vi "ConvertWaterMixValve4Calibration.vi"(8 "Water Mix Valve":u16(ring) items=["A1", "A2", "A3", "A4", "B1", "B2", "B3", "B4", "B5", "B6", "B7", "B8", "A5", "A6", "A7", "A8"], 9 "Ctr Water Valve":u16(ring) items=["A1", "A2", "A3", "A4", "B1", "B2", "B3", "B4", "B5", "B6", "B7", "B8", "A5", "A6", "A7", "A8"], 11 "Calibration Refs":T2) -> (0 "Water Calibration?":bool[](array[boolean]), 1 "PressList":u8[](array[numeric]), 2 "RatioList":dbl[](array[numeric]), 3 "Valve Signal Array":T1(array[cluster]))   [LabVIEW 2016]
uses:
  <vilib>/imath/engines/lvmath/Plug In/_Char/NIMS_CH_character datatype.ctl
  <vilib>/imath/engines/lvmath2/RunTimeEngine/VariableToken/Support/NIMS_Vector Boolean Index to I32 Index.vi
  <vilib>/imath/engines/lvmath2/RunTimeEngine/IndexRead/NIMS V(V).vi
  <instcachedir>/0/NIMS V(V)_298D9CB7BFEB42B8BC8D9C3C28AE8C70.lvgen/NIMS V(V)_298D9CB7BFEB42B8BC8D9C3C28AE8C70_001.vi
  <vilib>/imathl/engines/lvmath/Functions/Error Handling/Create Error.vi
  <instcachedir>/0/NIMS V(V)_298D9CB7BFEB42B8BC8D9C3C28AE8C70.lvgen/NIMS V(V)_298D9CB7BFEB42B8BC8D9C3C28AE8C70_002.vi
  <vilib>/imath/engines/lvmath2/RunTimeEngine/IndexReplace/NIMS V(V)=V.vi
  <instcachedir>/0/NIMS V(V)=V_BE8E060C6E1D4A13ABFD54A163A3AD30.lvgen/NIMS V(V)=V_BE8E060C6E1D4A13ABFD54A163A3AD30_000.vi
  <vilib>/imath/engines/lvmath2/RunTimeEngine/ErrorHandling/NIMS_Create Error From Enums.vi
  <vilib>/imath/engines/lvmath2/RunTimeEngine/BuiltInFunctions/findnz/NIMS_[1o]_findnz(GRowV).vi
  <instcachedir>/0/NIMS_[1o]_findnz(GRowV)_656056C849EF4762B1F0843BDDDEF2FF.lvgen/NIMS_[1o]_findnz(GRowV)_656056C849EF4762B1F0843BDDDEF2FF_000.vi
  <vilib>/imath/engines/lvmath/Plug In/_Char/NIMS_CH_Character RV to String.vi
  <vilib>/imath/engines/lvmath2/RunTimeEngine/BuiltInFunctions/length/NIMS_length(GV).vi
  <instcachedir>/0/NIMS_length(GV)_08A3D13377FD4E4B96F5795FBF3698FA.lvgen/NIMS_length(GV)_08A3D13377FD4E4B96F5795FBF3698FA_002.vi
  <vilib>/imath/engines/lvmath2/RunTimeEngine/BuiltInFunctions/random/NIMS_random.vi
  <vilib>/imath/engines/lvmath2/RunTimeSupport/NIMS_Error if Not Equal.vi
  <instcachedir>/0/NIMS_Error if Not Equal_EBDB539BFBF84063AF66BAE64AA6DE72.lvgen/NIMS_Error if Not Equal_EBDB539BFBF84063AF66BAE64AA6DE72_002.vi
  <vilib>/imath/engines/lvmath2/RunTimeEngine/IndexRead/NIMS V(M).vi
  <instcachedir>/0/NIMS V(M)_9C733378D59448EDB8B370EA0429D12A.lvgen/NIMS V(M)_9C733378D59448EDB8B370EA0429D12A_002.vi
  <instcachedir>/0/NIMS V(M)_9C733378D59448EDB8B370EA0429D12A.lvgen/NIMS V(M)_9C733378D59448EDB8B370EA0429D12A_001.vi
  <vilib>/imath/engines/lvmath2/RunTimeEngine/IndexReplace/NIMS V(V)=M.vi
  <instcachedir>/0/NIMS V(V)=M_4E1E70A83EF34EDC81D1F331EC25431D.lvgen/NIMS V(V)=M_4E1E70A83EF34EDC81D1F331EC25431D_001.vi
  <instcachedir>/0/NIMS V(M)_9C733378D59448EDB8B370EA0429D12A.lvgen/NIMS V(M)_9C733378D59448EDB8B370EA0429D12A_000.vi
  <instcachedir>/0/NIMS V(V)=M_4E1E70A83EF34EDC81D1F331EC25431D.lvgen/NIMS V(V)=M_4E1E70A83EF34EDC81D1F331EC25431D_002.vi
  <vilib>/imath/engines/lvmath2/RunTimeEngine/NodeEndStatement/NIMS_NodeEndStatement_Output.vi
  <instcachedir>/0/NIMS_NodeEndStatement_Output_53EC0D466D134D7ABD903AC30B43404B.lvgen/NIMS_NodeEndStatement_Output_53EC0D466D134D7ABD903AC30B43404B_013.vi
  <instcachedir>/0/NIMS_NodeEndStatement_Output_53EC0D466D134D7ABD903AC30B43404B.lvgen/NIMS_NodeEndStatement_Output_53EC0D466D134D7ABD903AC30B43404B_012.vi
  <instcachedir>/0/NIMS_NodeEndStatement_Output_53EC0D466D134D7ABD903AC30B43404B.lvgen/NIMS_NodeEndStatement_Output_53EC0D466D134D7ABD903AC30B43404B_011.vi
  <instcachedir>/0/NIMS_NodeEndStatement_Output_53EC0D466D134D7ABD903AC30B43404B.lvgen/NIMS_NodeEndStatement_Output_53EC0D466D134D7ABD903AC30B43404B_005.vi
  <vilib>/imath/engines/lvmath2/RunTimeEngine/ErrorHandling/NIMS_Finalize Error.vi
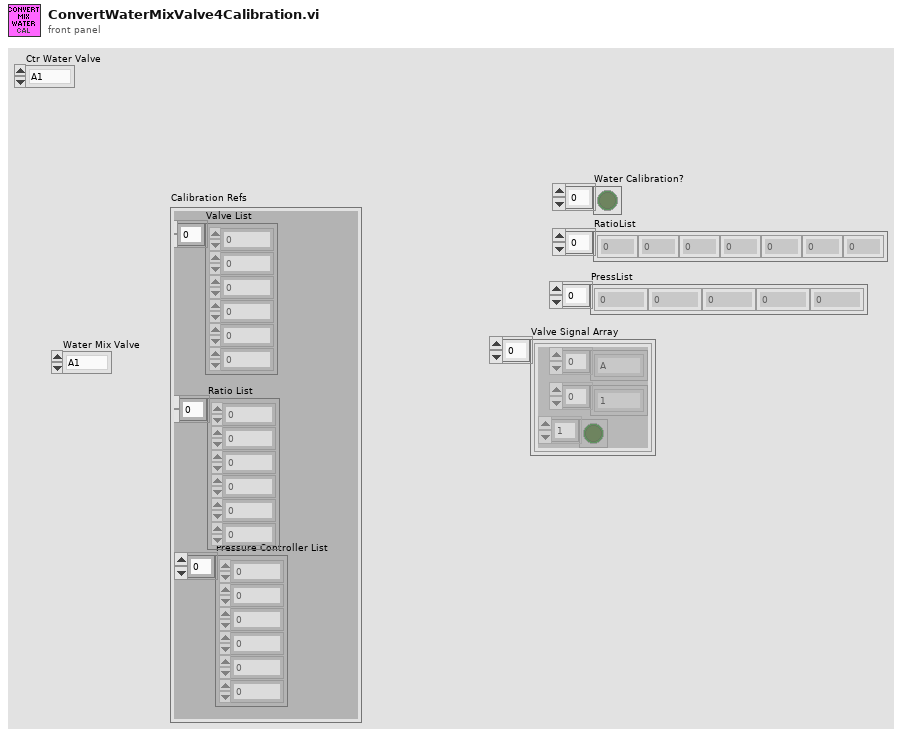
[diagram p1: front panel]
types:
  T1 = cluster{enum16{"A", "B", "C"}[], enum16{"1", "2", "3", "4", "5", "6", "7", "8"}[], bool[]}[]
  T2 = cluster{"Pressure Controller List":u8[], "Ratio List":dbl[], "Valve List":u16[]}
  T3 = cluster{"Flowboards":enum16{"A", "B", "C"}[], "Channels":enum16{"1", "2", "3", "4", "5", "6", "7", "8"}[], "States":bool[]}[]
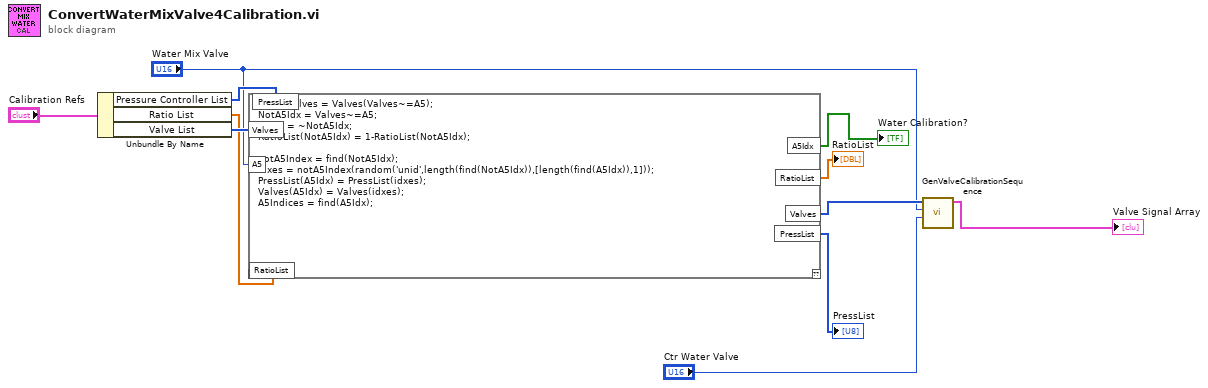
[diagram p0: block diagram]
diagram:
  n1 = Unbundle By Name("Calibration Refs") -> ("Pressure Controller List"=w10:u8[], "Ratio List"=w8:dbl[], "Valve List"=w9:u16[])
  n2 = mathscript code="NotA5Valves = Valves(Valves~=A5);\nNotA5Idx = Valves~=A5;\nA5Idx = ~NotA5Idx;\nRatioList(NotA5Idx) = 1-RatioList(NotA5Idx);\n\nnotA5Index = find(NotA5Idx);\nidxes = notA5Index(random('unid',length(find(NotA5Idx)),[length(find(A5Idx)),1]));\nPressList(A5Idx) = PressList(idxes);\nValves(A5Idx) = Valves(idxes);\nA5Indices = find(A5Idx);"("A5"="Water Mix Valve", "Valves"=w9, "PressList"=w10, "RatioList"=w8) -> ("RatioList"=→"RatioList":dbl[], "Valves"=w4:u16[], "PressList"=→"PressList":u8[], "A5Idx"=→"Water Calibration?":bool[])  [unwired: 1 in, 1 out]
  n3 = call "GenValveCalibrationSequence.vi"("Ctr Odor Valve"="Ctr Water Valve", "Water Mix Valve"="Water Mix Valve", "Valve List"=w4) -> ("Valve Sequence Array"=→"Valve Signal Array":T3)  [unwired: 8 in]
